vi "userauth_list.vi"() -> ()   [LabVIEW 2013]
doc: "Illustrates how to get the supported authentication methods."
uses:
  libssh2/libssh2_init_default.vi
  libssh2/libssh2_session_handshake_tcp.vi
  libssh2/libssh2.lvlib
panel:
  out "supported authentication schemes":string
  in  "username":string
  in  "hostname":string="localhost"
  out "error out":errorcluster
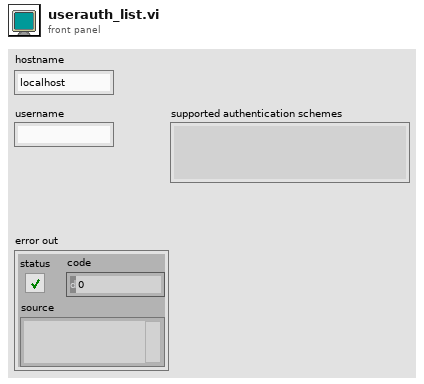
[diagram p1: front panel]
types:
  T1 = typedef "libssh2.lvlib/Session Refnum.ctl" = refnum<k1>
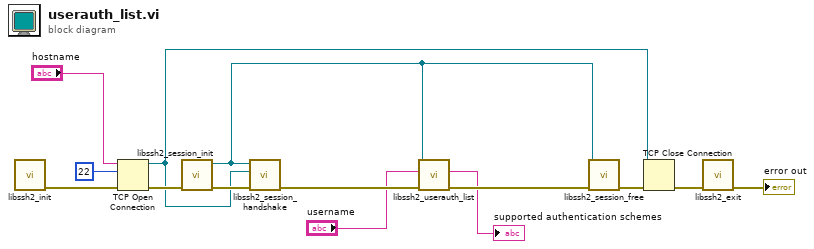
[diagram p0: block diagram]
diagram:
  n1 = call-poly "libssh2_init.vi"() -> ("error out"=w14:errorcluster)  [unwired: 11 in]
  n2 = TCP Open Connection(address="hostname", remote port or service name=u16 22, error in (no error)=w14) -> (connection ID=w6:refnum<k5>, error out=w7:errorcluster)  [unwired: 2 in]
  n3 = call "libssh2_session_init.vi"("error in (no error)"=w7) -> ("error out"=w9:errorcluster, "session"=w3:T1)  [unwired: 9 in]
  n4 = call-poly "libssh2_session_handshake.vi"("error in (no error)"=w9, "tcp connection"=w6, "session"=w3) -> ("error out"=w5:errorcluster)  [unwired: 8 in]
  n5 = call "libssh2_userauth_list.vi"("error in (no error)"=w5, "username"="username", "session"=w3) -> ("error out"=w4:errorcluster, "supported authentication schemes"=→"supported authentication schemes":string)  [unwired: 7 in]
  n6 = call "libssh2_session_free.vi"("error in (no error)"=w4, "session"=w3) -> ("error out"=w8:errorcluster)  [unwired: 9 in]
  n7 = TCP Close Connection(connection ID=w6, error in (no error)=w8) -> (error out=w11:errorcluster)  [unwired: 1 in, 1 out]
  n8 = call "libssh2_exit.vi"("error in (no error)"=w11) -> ("error out"=→"error out":errorcluster)  [unwired: 10 in]
